vi "laser_ideas.vi"() -> ()   [LabVIEW 2019]
uses:
  <vilib>/addons/control/pid/pid.llb/PID (DBL).vi
  <vilib>/addons/control/pid/NI_PID_pid.lvlib
panel:
  out "calc'd pid gains standard":T1
  out "dt out (s)":dbl format="%.3f"
  out "Waveform Chart":cluster{"Plant Output":dbl, "output":dbl}(graph)
  in  "stop":bool
  in  "pid gains ||":cluster{"Kp":dbl, "Ki":dbl, "Kd":dbl}={"Kp"=50.0, "Ki"=5000.0, "Kd"=0.0}
  in  "low sp":dbl format="%.2f"
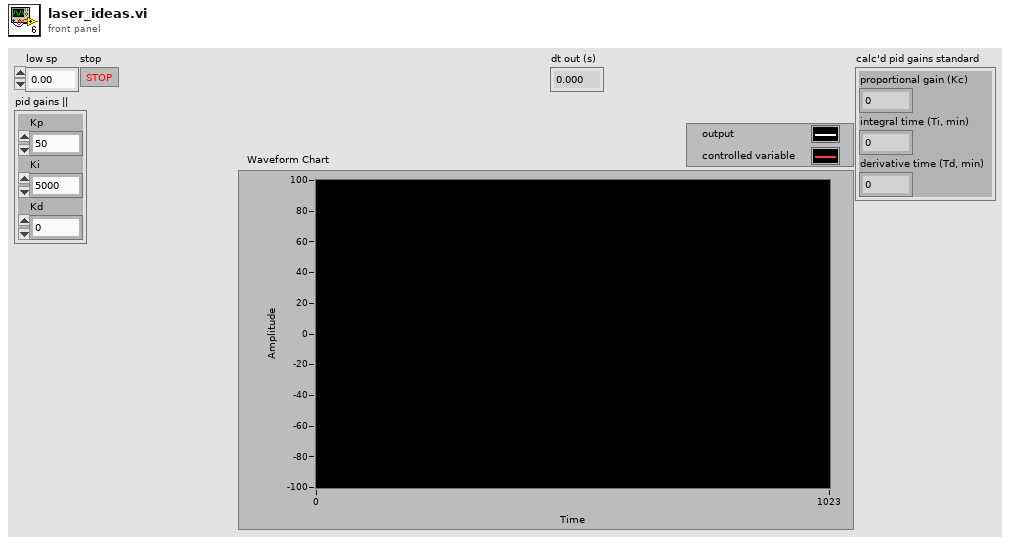
[diagram p1: front panel]
types:
  T1 = cluster{"proportional gain (Kc)":dbl, "integral time (Ti, min)":dbl, "derivative time (Td, min)":dbl}
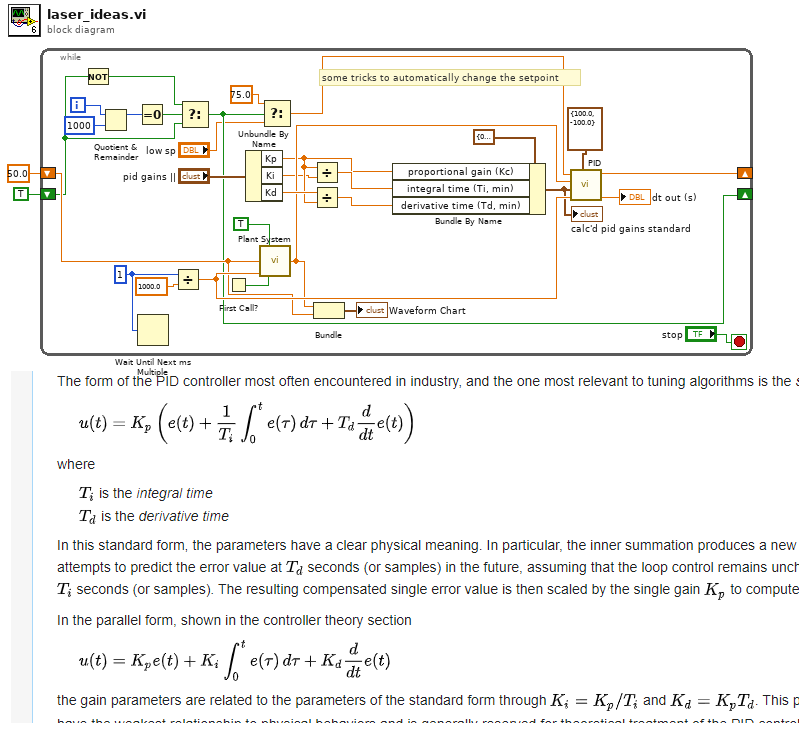
[diagram p0: block diagram]
diagram:
  n1 = while {
    shift-right: [w26] -> _
    shift-left: 50.0 ("output") -> [w22]
    shift-right: [w8] -> _
    shift-left: TRUE -> [w9]
    i -> [w15]
    stop <- "stop" stop-if-true
    w28 = u32 1 ("millisecond multiple")
    # "some tricks to automatically change the setpoint"
    n2 = Not(x=w9) -> (.not. x?=w10:bool)
    n3 = Quotient & Remainder(x=w15, y=1000) -> (x-y*floor(x/y)=w13:i32)  [unwired: 1 out]
    n4 = Equal To 0?(x=w13) -> (x = 0?=w11:bool)
    n5 = Wait Until Next ms Multiple(millisecond multiple=w28) -> ()  [unwired: 1 out]
    n6 = Divide(x=w28, y=1000.0) -> (x/y=w25:dbl)
    n7 = Select(t=w10, s=w11, f=w9) -> (s? t:f=w8:bool)
    n8 = First Call?() -> (First Call?: T/F=w20:bool)
    n9 = Unbundle By Name("pid gains ||") -> ("Kp"=w17:dbl, "Ki"=w16:dbl, "Kd"=w30:dbl)
    n10 = call "Plant System.vi"("Integrator ?"=TRUE, "Plant Input"=w22, "dt (s)"=w25, "reinitialize? (F)"=w20) -> ("Plant Output"=w21:dbl)  [unwired: 11 in]
    n11 = Select(t=75.0, s=w8, f="low sp") -> (s? t:f=w5:dbl)
    n12 = Divide(x=w17, y=w16) -> (x/y=w31:dbl)
    n13 = Divide(x=w30, y=w17) -> (x/y=w23:dbl)
    n14 = Bundle("Plant Output"=w21, "output"=w22) -> (→"Waveform Chart":cluster{"Plant Output":dbl, "output":dbl})  [unwired: 1 in]
    n15 = Bundle By Name(cluster=T1 {"proportional gain (Kc)"=0.0, "integral time (Ti, min)"=0.0, "derivative time (Td, min)"=0.0} ("pid gains standard"), "proportional gain (Kc)"=w17, "integral time (Ti, min)"=w31, "derivative time (Td, min)"=w23) -> (w3:T1)
    "calc'd pid gains standard" <- w3
    n16 = call-poly <vilib>:"PID.vi"("output range"=cluster{"output high":dbl, "output low":dbl} {"output high"=100.0, "output low"=-100.0}, "dt (s)"=w25, "PID gains"=w3, "process variable"=w21, "setpoint"=w5) -> ("dt out (s)"=→"dt out (s)":dbl, "output"=w26:dbl)  [unwired: 5 in]
  }
